vi "Select_ini.vi"(8 "error in":errorcluster, 10 "OS Specific path":T1(array[cluster]), 11 "OS Name":string) -> (0 "error out":errorcluster, 3 "OS Apecific INI":string)   [LabVIEW 2015]
panel:
  out "Number of OS Files":i32
  # "Select the scipt OS Wise"
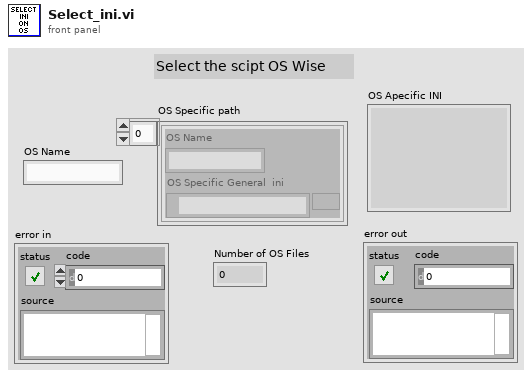
[diagram p1: front panel]
types:
  T1 = cluster{"OS Name":string, "OS Specific General  ini":path}[]
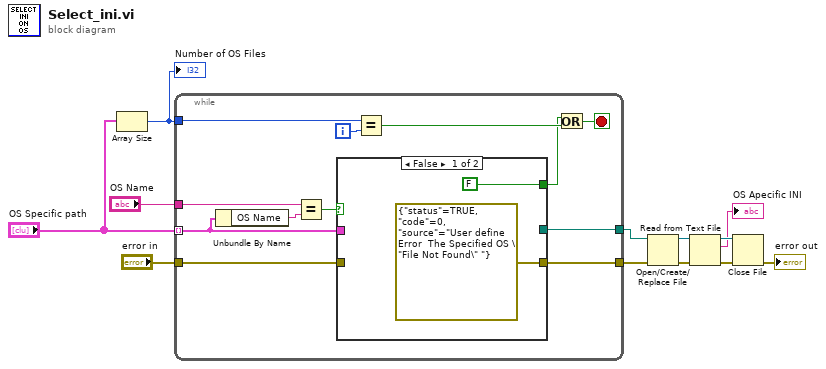
[diagram p0: block diagram]
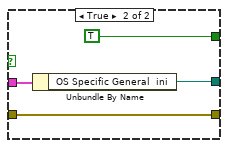
[diagram p2: hidden frame]
diagram:
  n1 = Array Size(array="OS Specific path") -> (size(s)=w1:i32)
  "Number of OS Files" <- w1
  n2 = while {
    tunnel: "OS Specific path" -> [w21] mode=indexing
    tunnel: "OS Name" -> [w23]
    tunnel: [w20] -> w4
    tunnel: [w19] -> w3
    tunnel: "error in" -> [w18]
    tunnel: w1 -> [w16]
    i -> [w17]
    stop <- w13 stop-if-true
    n3 = Unbundle By Name(w21) -> ("OS Name"=w24:string)
    n4 = Equal?(x=w23, y=w24) -> (x = y?=w22:bool)
    n5 = case shown="False" w22 {
      tunnel: w21 -> [_ w30]
      tunnel: [_ w29] -> w20
      tunnel: [errorcluster {"status"=TRUE, "code"=0, "source"="User define Error  The Specified OS \"File Not Found\" "} ("error in") w28] -> w19
      tunnel: w18 -> [_ w28]
      tunnel: [FALSE TRUE] -> w14
      frame False {
      }
      frame True {
        n6 = Unbundle By Name(w30) -> ("OS Specific General  ini"=w29:path)
      }
    }
    n7 = Equal?(x=w16, y=w17) -> (x = y?=w15:bool)
    n8 = Or(x=w14, y=w15) -> (x .or. y?=w13:bool)
  }
  n9 = Open/Create/Replace File(file path (use dialog)=w4, error in=w3) -> (refnum out=w12:refnum<file>, error out=w10:errorcluster)  [unwired: 4 in, 1 out]
  n10 = Read from Text File(file (use dialog)=w12, error in=w10) -> (refnum out=w11:refnum<file>, text=→"OS Apecific INI":string, error out=w9:errorcluster)  [unwired: 2 in, 1 out]
  n11 = Close File(refnum=w11, error in=w9) -> (error out=→"error out":errorcluster)  [unwired: 1 out]
